vi "Poly_One_Numb_Get.vi"(8 "error in":errorcluster, 9 "Button 2 Text":string, 10 "Button 1 Text":string, 11 "Message":string) -> (0 "error out":errorcluster, 2 "Text Out":u32 caption="Input Text", 3 "Indicator 1":bool)   [LabVIEW 2024, in "Launcher_DTU.lvlib"]
uses:
  Launcher_DTU.lvlib
panel:
  in  "Text":u32 caption="Input Text"
  out "Message":string
  in  "Button 2":bool
  in  "Button 1":bool
  # "User Input"
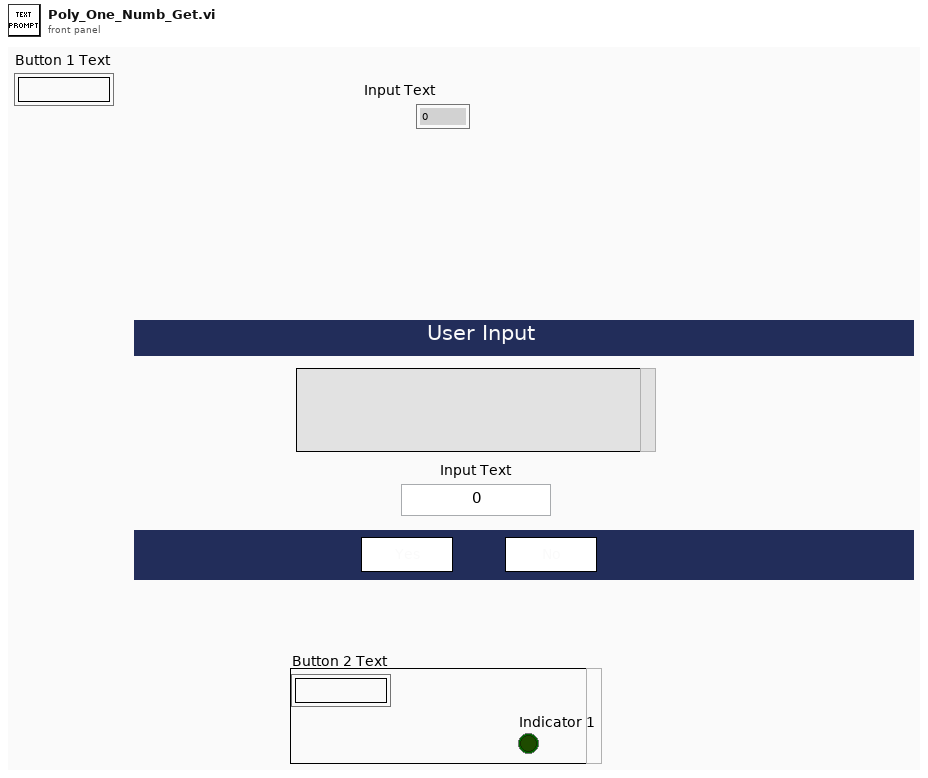
[diagram p1: front panel]
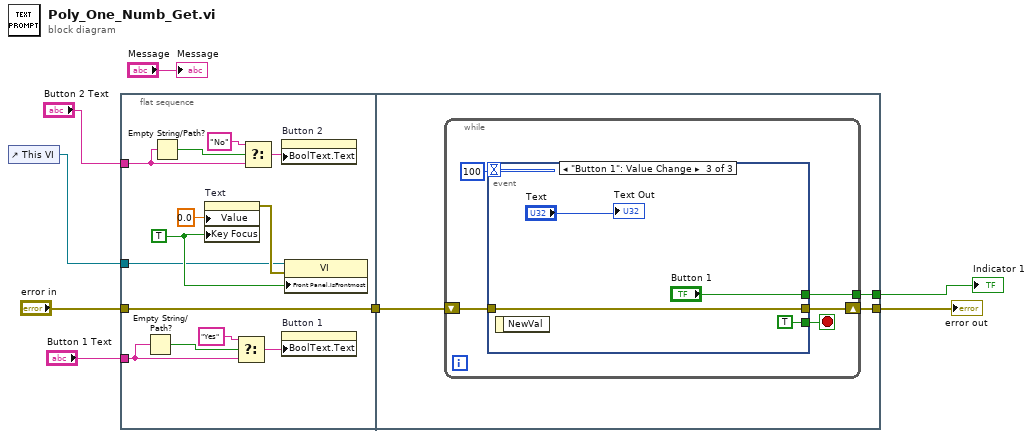
[diagram p0: block diagram]
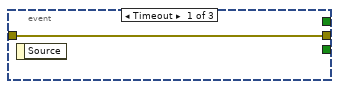
[diagram p2: hidden frame]
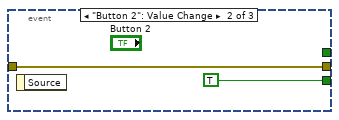
[diagram p3: hidden frame]
diagram:
  n1 = control-ref of="This VI"() -> (w1:refnum<vi>)
  n2 = flat-sequence {
    tunnel: [w21] -> w7
    tunnel: "error in" -> [w21]
    tunnel: "Button 1 Text" -> [w19]
    tunnel: "Button 2 Text" -> [w13]
    tunnel: w1 -> [w10]
    tunnel: [w24] -> w8
    tunnel: w7 -> [w23]
    tunnel: [w22] -> w4
    frame #0 {
      w11 = TRUE ("Key Focus")
      n3 = Empty String/Path?(string/path=w19) -> (empty?=w20:bool)
      n4 = Empty String/Path?(string/path=w13) -> (empty?=w15:bool)
      n5 = property on="Text" class="DigNum (strict)"("Value"=0.0 ("Text"), "Key Focus"=w11) -> (error out=w12:errorcluster)  [unwired: 2 in, 1 out]
      n6 = Select(t="Yes", s=w20, f=w19) -> (s? t:f=w18:string)
      n7 = Select(t="No", s=w15, f=w13) -> (s? t:f=w14:string)
      n8 = property on="Button 2" class="Bool"("BoolText.Text"=w14) -> ()  [unwired: 2 in, 2 out]
      n9 = property on="Button 1" class="Bool"("BoolText.Text"=w18) -> ()  [unwired: 2 in, 2 out]
      n10 = property class="VI"(reference=w10, error in=w12, "Front Panel.IsFrontmost"=w11) -> ()  [unwired: 2 out]
    }
    frame #1 {
      n11 = while {
        shift-right: [w27] -> w24
        shift-left: w23 -> [w28]
        tunnel: [w26] -> w22
        stop <- w25 stop-if-true
        n12 = event shown="[2] \"Button 1\": Value Change" {
          selector: _ -> [_ _ _]
          dyn-events: _ -> [_ _ _]
          timeout: 100 -> [_ _ _]
          tunnel: [_ TRUE TRUE] -> w25
          tunnel: w28 -> [w30 w32 w35]
          tunnel: [w30 w32 w35] -> w27
          tunnel: [_ _ "Button 1"] -> w26
          event Timeout {
            n13 = event-data() -> ()  [unwired: 1 in, 1 out]
          }
          event "Button 2": Value Change {
            n14 = event-data() -> ()  [unwired: 1 in, 1 out]
          }
          event "Button 1": Value Change {
            n15 = event-data() -> ()  [unwired: 1 in, 1 out]
            "Text Out" <- "Text"
          }
        }
      }
    }
  }
  "error out" <- w8
  "Indicator 1" <- w4
  "Message" <- "Message"
